vi "UMS.vi"() -> ()   [LabVIEW 2020]
uses:
  Machine.ctl
  Arrays.ctl
  Array.ctl
  Platter.ctl
panel:
  out "x+1":u64
  in  "Path":path=path "/Users/toshi/Documents/UM/9p.um"
  out "output":string
  in  "input":string="(\\b.bb)(\\v.vv)06FHPVboundvarHRAk"
  out "read program":T1 format="%032b"
  in  "initial machine state":T3={"Arrays"={}, "Finger"=0, "Registers"=[0, 0, 0, 0, 0, 0, 0, 0], "next id"=1} {"Registers" format="%032b"; "Arrays"."Array" format="%032b"}
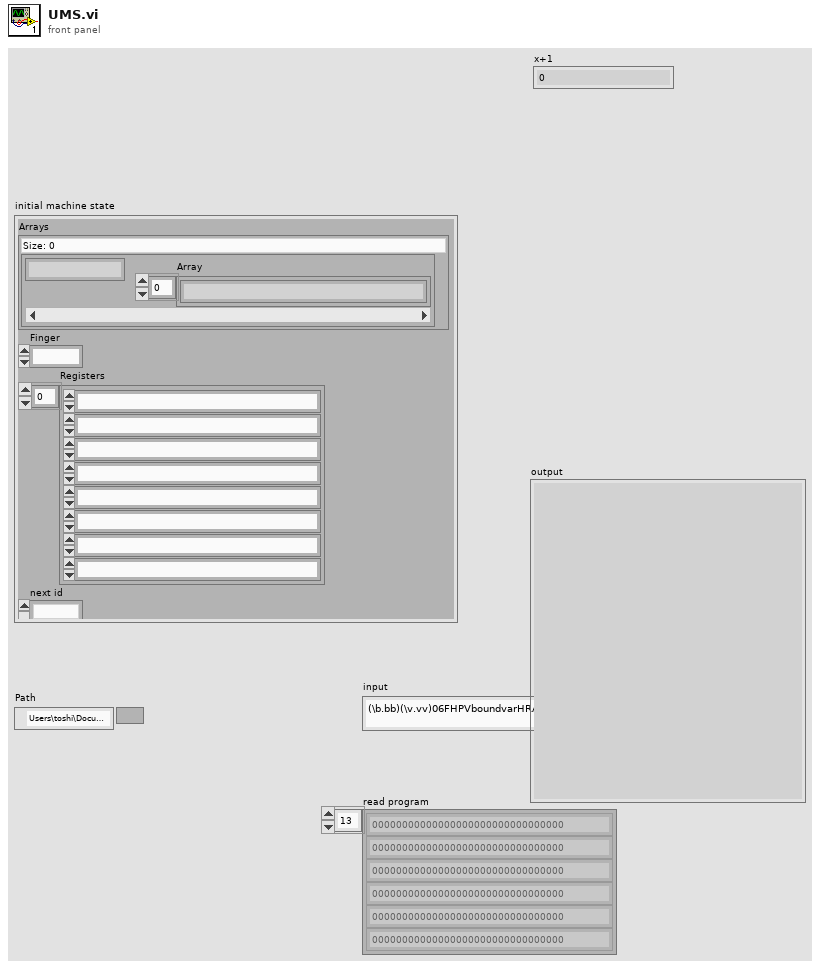
[diagram p1: front panel]
types:
  T1 = typedef "Array.ctl" = T2[]
  T2 = typedef "Platter.ctl" = u32
  T3 = typedef "Machine.ctl" = cluster{"Arrays":T4, "Finger":u32, "Registers":T2[], "next id":u32}
  T4 = typedef "Arrays.ctl" = map{string, T1}
  T5 = enum16{"big-endian, network order", "native, host order", "little-endian"}
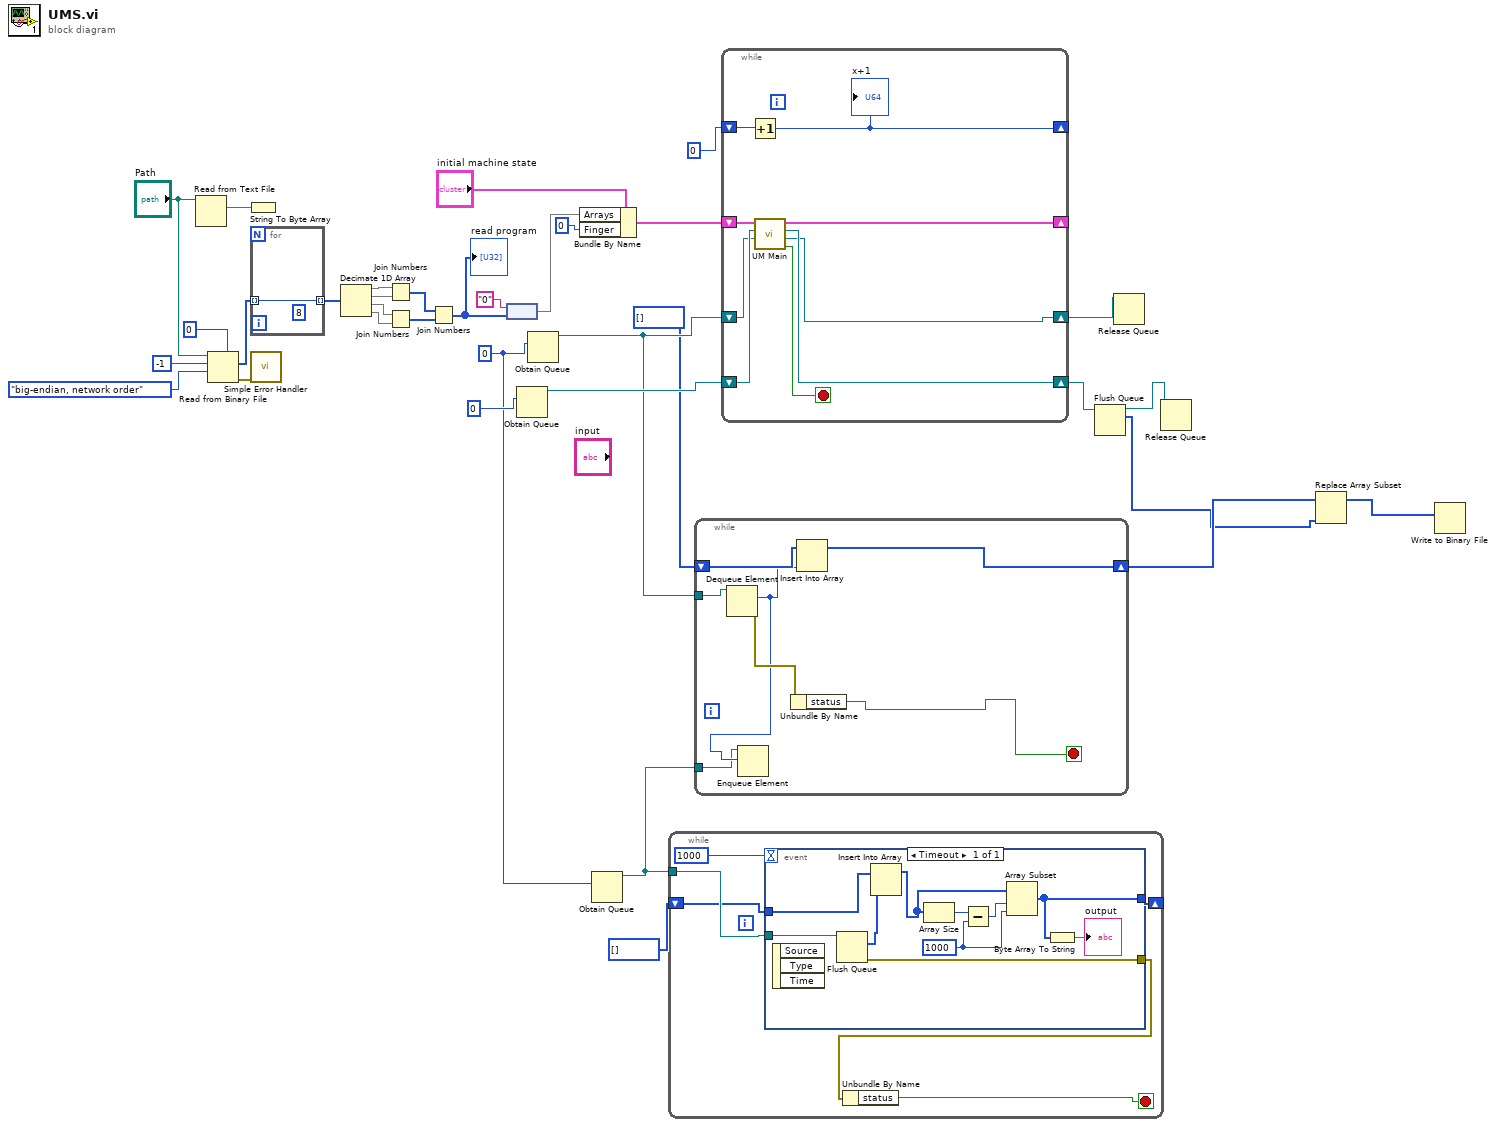
[diagram p0: block diagram]
diagram:
  w3 = u8 0
  n1 = Read from Text File(file (use dialog)="Path") -> (text=w20:string)  [unwired: 3 in, 3 out]
  n2 = Read from Binary File(5:u8 0, 9:T5."big-endian, network order" ("byte order (0:big-endian, network order)"), 10:-1 ("count (1)"), 11:"Path") -> (0:w22:errorcluster, 2:w17:u8[])  [unwired: 2 in, 2 out]
  n3 = String To Byte Array(string=w20) -> ()  [unwired: 1 out]
  n4 = for {
    tunnel: w17 -> [w35] mode=indexing
    tunnel: [w35] -> w16 mode=indexing
    (unwired) 8
  }
  n5 = call <vilib>:"Simple Error Handler.vi"("error in (no error)"=w22) -> ()  [unwired: 4 in, 5 out]
  n6 = Decimate 1D Array(w16) -> (w29:u8[], w30:u8[], w31:u8[], w32:u8[])
  n7 = Join Numbers(hi=w29, lo=w30) -> ((hi.lo)=w33:u16[])
  n8 = Join Numbers(hi=w31, lo=w32) -> ((hi.lo)=w34:u16[])
  n9 = Join Numbers(hi=w33, lo=w34) -> ((hi.lo)=w27:u32[])
  "read program" <- w27
  n10 = node("0" ("key"), w27) -> (w26:map{string, u32[]})
  n11 = Obtain Queue(element data type=u8 0) -> (queue out=w13:refnum<queue>)  [unwired: 4 in, 2 out]
  n12 = Obtain Queue(element data type=w3) -> (queue out=w11:refnum<queue>)  [unwired: 4 in, 2 out]
  n13 = Bundle By Name(cluster="initial machine state", "Arrays"=w26, "Finger"=u32 0) -> (w23:T3)
  n14 = Obtain Queue(element data type=w3) -> (queue out=w5:refnum<queue>)  [unwired: 4 in, 2 out]
  n15 = while {
    tunnel: w5 -> [w41]
    shift-right: [w38] -> _
    shift-left: u8[] [] -> [w40]
    stop <- w36 stop-if-true
    n16 = event shown="[0] Timeout" {
      selector: _ -> [_]
      dyn-events: _ -> [_]
      timeout: 1000 -> [_]
      tunnel: w41 -> [w50]
      tunnel: w40 -> [w44]
      tunnel: [w46] -> w38
      tunnel: [w45] -> w37
      event Timeout {
        w47 = 1000 ("y")
        n17 = event-data() -> ()  [unwired: 1 in, 3 out]
        n18 = Flush Queue(queue=w50) -> (remaining elements=w43:u8[], error out=w45:errorcluster)  [unwired: 1 in, 1 out]
        n19 = Insert Into Array(array=w44, new element=w43) -> (w42:u8[])  [unwired: 1 in]
        n20 = Array Size(array=w42) -> (size(s)=w49:i32)
        n21 = Subtract(x=w49, y=w47) -> (x-y=w48:i32)
        n22 = Array Subset(array=w42, index=w48, length=w47) -> (w46:u8[])
        n23 = Byte Array To String(unsigned byte array=w46) -> (string=→"output":string)
      }
    }
    n24 = Unbundle By Name(w37) -> ("status"=w36:bool)
  }
  n25 = while {
    shift-right: [w54] -> w8
    shift-left: u8[] [] -> [w58]
    tunnel: w11 -> [w57]
    tunnel: w5 -> [w52]
    stop <- w55 stop-if-true
    n26 = Dequeue Element(queue=w57) -> (element=w53:u8, error out=w56:errorcluster)  [unwired: 2 in, 2 out]
    n27 = Enqueue Element(queue=w52, element=w53) -> ()  [unwired: 2 in, 3 out]
    n28 = Unbundle By Name(w56) -> ("status"=w55:bool)
    n29 = Insert Into Array(array=w58, new element=w53) -> (w54:u8[])  [unwired: 1 in]
  }
  n30 = while {
    shift-right: [w66] -> _
    shift-left: w23 -> [w67]
    shift-right: [w61] -> w12
    shift-left: w11 -> [w64]
    shift-right: [w63] -> w10
    shift-left: w13 -> [w65]
    shift-right: [w59] -> _
    shift-left: u64 0 -> [w60]
    stop <- w62 stop-if-true
    n31 = Increment(x=w60) -> (x+1=w59:u64)
    "x+1" <- w59
    n32 = call "UM Main.vi"("output in"=w64, "input in"=w65, "machine in"=w67) -> ("terminate"=w62:bool, "output out"=w61:refnum<queue>, "input out"=w63:refnum<queue>, "machine out"=w66:T3)  [unwired: 3 in]
  }
  n33 = Flush Queue(queue=w10) -> (queue out=w9:refnum<queue>, remaining elements=w7:u8[])  [unwired: 1 in, 1 out]
  n34 = Release Queue(queue=w12) -> ()  [unwired: 2 in, 3 out]
  n35 = Release Queue(queue=w9) -> ()  [unwired: 2 in, 3 out]
  n36 = Replace Array Subset(array=w8, new element=w7) -> (w6:u8[])  [unwired: 1 in]
  n37 = Write to Binary File(data=w6) -> ()  [unwired: 5 in, 3 out]
